vi "output-frame.vi"(8 "error in (no error)":errorcluster, 9 "CAN frame":T1 {"payload" format="%x"; "timestamp" format="%<%.7X\n%x>T"; "type" items=["CAN Data"=0, "CAN Remote"=1, "CAN Bus Error"=2, "J1939 Data"=192, "Delay"=224, "Log Trigger"=225, "Start Trigger"=226]; "identifier" format="%x"}, 11 "fi in":refnum<class "bFrameIO.lvclass">) -> (0 "error out":errorcluster, 3 "fi out":refnum<class "bFrameIO.lvclass">)   [LabVIEW 2015, in "bFrameIO.lvclass"]
uses:
  bFrameIO.lvclass
  <vilib>/xnet/xnet.llb/XNET Frame CAN.ctl
  <vilib>/xnet/xnet.llb/XNET Frame Type CAN.ctl
  bFrameIO.lvclass/bFrameIO.ctl
  read-baud-rate.vi
  read-device.vi
  <vilib>/xnet/xnet.llb/XNET String To IO Name (Frame).vi
  <vilib>/xnet/xnet.llb/XNET Create Session (Frame Output Single-point).vi
  <vilib>/xnet/xnet.llb/XNET Write (Frame CAN).vi
  class.can.table/bAPPdata.lvclass
  <resource>/objmgr/xnet.rc
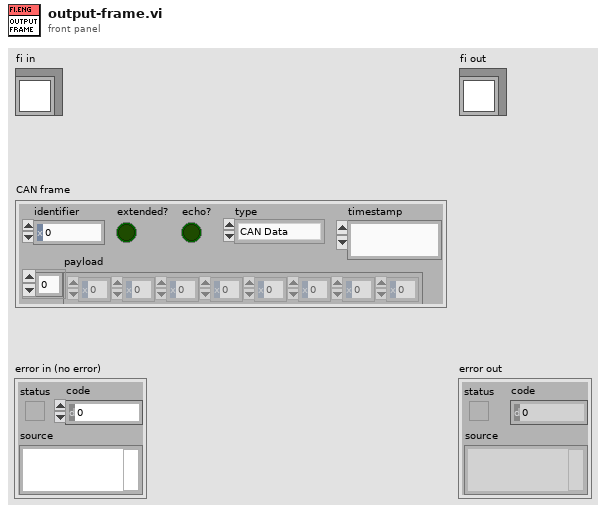
[diagram p1: front panel]
types:
  T1 = typedef "XNET Frame CAN.ctl" = cluster{"timestamp":timestamp, "payload":u8[], "identifier":u32, "type":T2, "extended?":bool, "echo?":bool}
  T2 = typedef "XNET Frame Type CAN.ctl" = u8
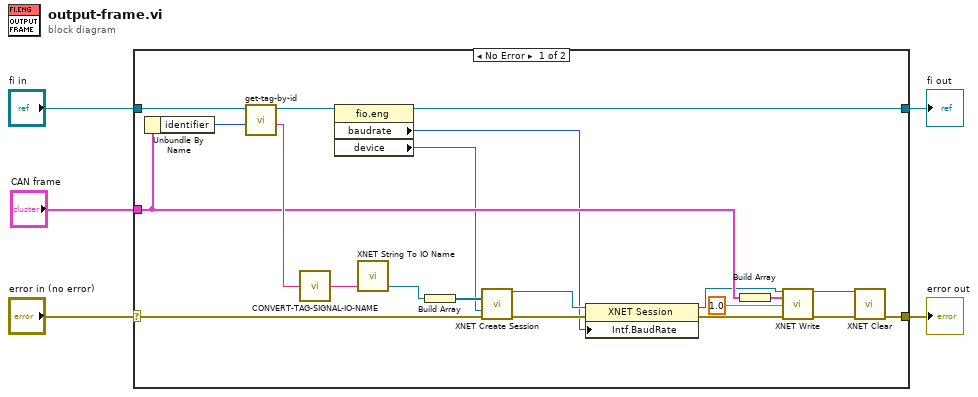
[diagram p0: block diagram]
diagram:
  n1 = case shown="No Error" "error in (no error)" {
    selector: "error in (no error)" -> [w25 w28]
    tunnel: [w22 w28] -> w4
    tunnel: [w8 w27] -> w2
    tunnel: "fi in" -> [w26 w27]
    tunnel: "CAN frame" -> [w14 _]
    frame No Error {
      n2 = Unbundle By Name(w14) -> ("identifier"=w13:u32)
      n3 = call "get-tag-by-id.vi"("id"=w13, "CANtable in"=w26) -> ("tag"=w15:string, "CANtable out"=w17:refnum<class "bFrameIO.lvclass">)  [unwired: 7 in, 1 out]
      n4 = call "CONVERT-TAG-SIGNAL-IO-NAME.vi"("tag"=w15) -> ("signal"=w16:string)  [unwired: 4 in]
      n5 = property class="fio.eng"(reference=w17) -> (reference out=w8:refnum<class "bFrameIO.lvclass">, "baudrate"=w6:u32, "device"=w7:refnum<k21>)  [unwired: 1 in, 1 out]
      n6 = call-poly <vilib>:"XNET String To IO Name.vi"("string"=w16) -> ("XNET Frame"=w19:refnum<k21>)  [unwired: 4 out]
      n7 = Build Array(w19) -> (w18:refnum<k21>[])
      n8 = call-poly <vilib>:"XNET Create Session.vi"("frame list"=w18, "interface"=w7, "error in (no error)"=w25) -> ("session out"=w10:refnum<k21>, "error out"=w12:errorcluster)  [unwired: 11 in]
      n9 = property class="XNET Session"(reference=w10, error in=w12, "Intf.BaudRate"=w6) -> (reference out=w9:refnum<k21>, error out=w11:errorcluster)
      n10 = Build Array(w14) -> (w23:T1[])
      n11 = call-poly <vilib>:"XNET Write.vi"("session in"=w9, "data"=w23, "timeout (10)"=1.0, "error in (no error)"=w11) -> ("session out"=w21:refnum<k21>, "error out"=w24:errorcluster)  [unwired: 10 in]
      n12 = call <vilib>:"XNET Clear.vi"("session in"=w21, "error in (no error)"=w24) -> ("error out"=w22:errorcluster)  [unwired: 13 in]
    }
    frame Error {
    }
  }
  "error out" <- w4
  "fi out" <- w2
